vi "_Raise Nav Complete Event.vi"(4 "Display State In":T1, 5 "Event Data":cluster{"sender":refnum<k24>, "e":refnum<k24>}, 6 "Control Ref":refnum<k24>, 7 "Event Common Data":T2) -> ()   [LabVIEW 2020, in "WebView2 Control.xctl"]
uses:
  WebView2 Control.xctl
  E:/Labview/LV 2020/Libs/WebView2/LV-WebView2/Source/Libs/Microsoft.Web.WebView2.Core.dll
  Libs/Microsoft.Web.WebView2.Core.dll
  Events.ctl
  Navigation Event Data.ctl
  Source Changed Event Data.ctl
  Navigation Start Event Data.ctl
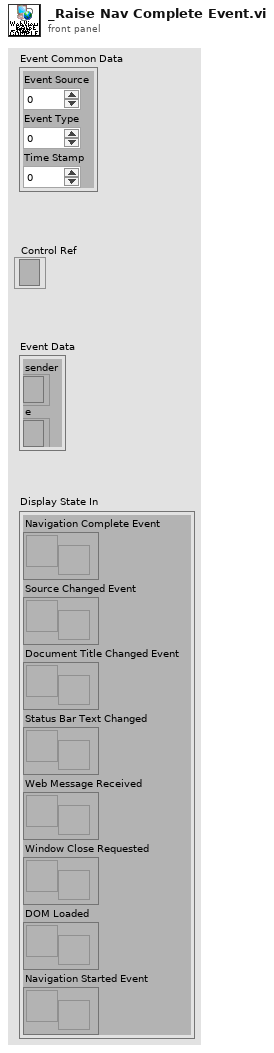
[diagram p1: front panel]
types:
  T1 = typedef "WebView2 Control.xctl/Events.ctl" = cluster{"Navigation Complete Event":refnum<user-event>, "Source Changed Event":refnum<user-event>, "Document Title Changed Event":refnum<user-event>, "Status Bar Text Changed":refnum<user-event>, "Web Message Received":refnum<user-event>, "Window Close Requested":refnum<user-event>, "DOM Loaded":refnum<user-event>, "Navigation Started Event":refnum<user-event>}
  T2 = cluster{"Event Source":i32, "Event Type":u32, "Time Stamp":u32}
  T3 = typedef "WebView2 Control.xctl/Navigation Event Data.ctl" = cluster{"HttpStatusCode":i32, "IsSuccess":bool, "NavigationId":u64, "WebErrorStatus":i32}
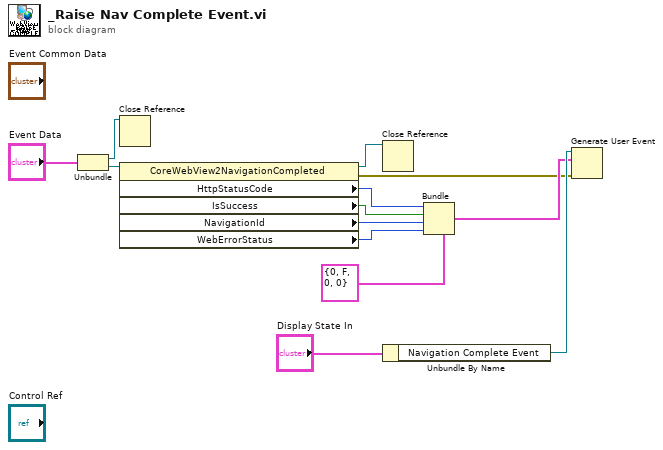
[diagram p0: block diagram]
diagram:
  n1 = Unbundle("Event Data") -> ("sender"=w2:refnum<k24>, "e"=w10:refnum<k24>)
  n2 = Close Reference(reference=w2) -> ()  [unwired: 1 in, 1 out]
  n3 = property class="CoreWebView2NavigationCompleted"(reference=w10) -> (reference out=w1:refnum<k24>, error out=w3:errorcluster, "HttpStatusCode"=w9:i32, "IsSuccess"=w8:bool, "NavigationId"=w7:u64, "WebErrorStatus"=w6:i32)  [unwired: 1 in]
  n4 = Close Reference(reference=w1) -> ()  [unwired: 1 in, 1 out]
  n5 = Unbundle By Name("Display State In") -> ("Navigation Complete Event"=w13:refnum<user-event>)
  n6 = Bundle(cluster=T3 {"HttpStatusCode"=0, "IsSuccess"=FALSE, "NavigationId"=0, "WebErrorStatus"=0} ("output cluster"), "HttpStatusCode"=w9, "IsSuccess"=w8, "NavigationId"=w7, "WebErrorStatus"=w6) -> (w4:T3)
  n7 = Generate User Event(user event=w13, event data cluster=w4, error in=w3) -> ()  [unwired: 1 in, 2 out]
